vi "test_libssh2_channel_send_eof.vi"() -> ()   [LabVIEW 2017, in "integration_tests.lvlib"]
uses:
  integration_tests.lvlib
  libssh2/libssh2_channel_open_ex.vi
  support/support.lvlib
  libssh2/libssh2.lvlib
  <vilib>/PNR/Transparent Assertions/Transparent Assertions/Transparent Assertions.lvlib
panel:
  out "error out":errorcluster
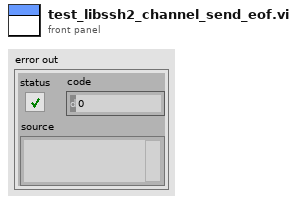
[diagram p1: front panel]
types:
  T1 = typedef "libssh2.lvlib/Session Refnum.ctl" = refnum<k1>
  T2 = typedef "libssh2.lvlib/Channel Refnum.ctl" = refnum<k1>
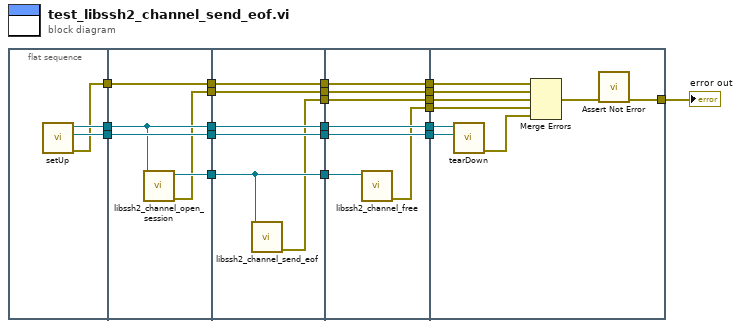
[diagram p0: block diagram]
diagram:
  n1 = flat-sequence {
    tunnel: [w24] -> w21
    tunnel: [w23] -> w20
    tunnel: [w22] -> w19
    tunnel: w21 -> [w28]
    tunnel: w20 -> [w29]
    tunnel: [w28] -> w7
    tunnel: [w29] -> w6
    tunnel: [w27] -> w5
    tunnel: w19 -> [w26]
    tunnel: [w26] -> w4
    tunnel: [w25] -> w3
    tunnel: w7 -> [w35]
    tunnel: [w35] -> w12
    tunnel: w6 -> [w34]
    tunnel: [w34] -> w11
    tunnel: w4 -> [w33]
    tunnel: [w33] -> w10
    tunnel: w3 -> [w32]
    tunnel: [w32] -> w9
    tunnel: w5 -> [w31]
    tunnel: [w31] -> w8
    tunnel: [w30] -> w2
    tunnel: w12 -> [w42]
    tunnel: w11 -> [w41]
    tunnel: [w42] -> w18
    tunnel: [w41] -> w17
    tunnel: [w40] -> w16
    tunnel: w10 -> [w39]
    tunnel: [w39] -> w15
    tunnel: w9 -> [w38]
    tunnel: [w38] -> w14
    tunnel: w8 -> [w37]
    tunnel: w2 -> [w36]
    tunnel: [w36] -> w1
    tunnel: w18 -> [w51]
    tunnel: w17 -> [w50]
    tunnel: [w49] -> w13
    tunnel: w16 -> [w47]
    tunnel: w15 -> [w46]
    tunnel: w14 -> [w44]
    tunnel: w1 -> [w43]
    frame #0 {
      n2 = call "setUp.vi"() -> ("error out"=w22:errorcluster, "connection ID"=w23:refnum<k5>, "session"=w24:T1)  [unwired: 9 in]
    }
    frame #1 {
      n3 = call "libssh2_channel_open_session.vi"("session"=w28) -> ("error out"=w25:errorcluster, "channel"=w27:T2)  [unwired: 9 in]
    }
    frame #2 {
      n4 = call "libssh2_channel_send_eof.vi"("channel"=w31) -> ("error out"=w30:errorcluster)  [unwired: 10 in]
    }
    frame #3 {
      n5 = call "libssh2_channel_free.vi"("channel"=w37) -> ("error out"=w40:errorcluster)  [unwired: 10 in]
    }
    frame #4 {
      n6 = call "tearDown.vi"("connection ID"=w50, "session"=w51) -> ("error out"=w48:errorcluster)  [unwired: 9 in]
      n7 = Merge Errors(w46, w44, w43, w47, w48) -> (w45:errorcluster)
      n8 = call <vilib>:"Assert Not Error.vi"("error in (no error)"=w45) -> ("error out"=w49:errorcluster)  [unwired: 10 in]
    }
  }
  "error out" <- w13
